vi "read_input_data.vi"(5 "Modulation info":T1={"Fs full"=0.0, "Fs high"=0.0, "Fs low"=0.0, "Read size"=5000, "FFT size low"=5000, "df low"=5000.0, "High carriers"=[], "Low carriers"=[], "Hi channels at low"=[7]} {"Hi channels at low" min=0 step=1; "Low carriers" format="%#_6p"; "High carriers" format="%#_6p"}, 7 "Config":T2={"IO params"={"Conversion"={"Rate"=4.0, "In channels"=2, "Out channels"=4}, "Carriers"={"Phase shift"=180.0, "Levels"=[[0.8, 0.8, 0.8], [0.03, 0.03, 0.03]], "Delay samples"=73.15}}, "High rate STFT"={"Win param"=101.5, "Window type"=61, "Win order"=2, "DFT size"=64, "Channels"=[7], "Oversample"=64}, "Low rate STFT"={"Win param"=120.0, "Window type"=61, "Win order"=8, "DFT size"=64, "Channels"=[7], "Oversample"=64}, "Filtering"={"Hum"={"Frequency"=0.0, "Tc"=0.0, "Limit"=101.5, "FFT filter"=FALSE, "Detrend mode"=enum."Robust linear", "Enable"=FALSE}, "Kalman"={"Process noise"=101.5, "Measure noise"=101.5, "Unlock m noise"=101.5, "Mode"=enum."FFT"}, "Distortion"={"LF cut"=101.5, "Tc"=3.0, "Limit"=101.5, "FFT filter"=FALSE, "Detrend mode"=enum."Robust linear", "Enable"=FALSE}, "Lowpass"={"Frequency"=0.0, "Order"=0, "Enable"=FALSE}, "Impulse"={"Win order"=102, "Locked limit"=101.5, "Locked count"=102, "Threshold Tc"=101.5, "Thresh sigmas"=101.5, "Thresh min"=101.5, "After"=0, "Detrend"=FALSE, "Enable"=FALSE}}} {"Filtering"."Impulse"."Thresh min" format="%#_3p"; "Filtering"."Impulse"."Threshold Tc" format="%#_3p"; "Filtering"."Impulse"."Locked limit" format="%#_3p"; "Filtering"."Impulse"."Thresh sigmas" format="%#_3p"; "Filtering"."Lowpass"."Frequency" format="%#_4p"; "Filtering"."Distortion"."Limit" format="%#_3p"; "Filtering"."Distortion"."LF cut" format="%#_3p"; "Filtering"."Kalman"."Unlock m noise" format="%#_3p"; "Filtering"."Kalman"."Measure noise" format="%#_3p"; "Filtering"."Kalman"."Process noise" format="%#_3p"; "Filtering"."Hum"."Limit" format="%#_3p"; "Filtering"."Hum"."Frequency" format="%#_4p"; "Low rate STFT"."Oversample" min=1 step=1; "Low rate STFT"."Channels" min=0 step=1; "Low rate STFT"."DFT size" min=1 step=1; "Low rate STFT"."Window type" items=["Rectangle"=0, "Hanning"=1, "Hamming"=2, "Blackman-Harris"=3, "Exact Blackman"=4, "Blackman"=5, "Flat Top"=6, "4 Term B-Harris "=7, "7 Term B-Harris"=8, "Low Sidelobe"=9, "Blackman Nuttall"=11, "Triangle"=30, "Bartlett-Hanning"=31, "Bohman"=32, "Parzen"=33, "Welch"=34, "Kaiser"=60, "Dolph-Chebyshev"=61, "Gaussian"=62]; "High rate STFT"."Oversample" min=1 step=1; "High rate STFT"."Channels" min=0 step=1; "High rate STFT"."DFT size" min=1 step=1; "High rate STFT"."Window type" items=["Rectangle"=0, "Hanning"=1, "Hamming"=2, "Blackman-Harris"=3, "Exact Blackman"=4, "Blackman"=5, "Flat Top"=6, "4 Term B-Harris "=7, "7 Term B-Harris"=8, "Low Sidelobe"=9, "Blackman Nuttall"=11, "Triangle"=30, "Bartlett-Hanning"=31, "Bohman"=32, "Parzen"=33, "Welch"=34, "Kaiser"=60, "Dolph-Chebyshev"=61, "Gaussian"=62]; "IO params"."Carriers"."Levels" min=0.0 step=0.1; "IO params"."Conversion"."Rate" format="%#_8g"}, 8 "error in":errorcluster, 9 "TCP channels":u32=3 min=1 max=12) -> (0 "error out":errorcluster, 1 "Data":i32[][](array[numeric]) format="%8x", 4 "TCP input":bool)   [LabVIEW 2014]
uses:
  ilemt_config.ctl
  IO_params.ctl
  stft_params.ctl
  <vilib>/Analysis/4window.llb/windowTd.ctl
  filter_params.ctl
  detrend_mode.ctl
  modulation_info.ctl
  ilemt_globals.vi
  <vilib>/Analysis/NI_AALPro.lvlib
panel:
  in  "Diff tag":u32 min=1 max=12
  in  "Same tag":u32 min=1 max=12
  out "Data size":i32[](array[numeric])
  out "length":i32
  in  "Timeouts":i32
  in  "Close count":i32
  out "error IO":errorcluster
  in  "TCP timeout ms":i32=5000
  # "Read the input data using TCP"
  # "Data read. Each row is data for one input channel.   Data is integer fraction of Bits/sample.  Eg. if bits/sample is 32, then data range is +/- 2^31, regardless of actual ADC resolution (in other words the data is low padded with zeros)."
  # "Number of channels to read"
  # "Did we read input from TCP?"
  # "Locals:"
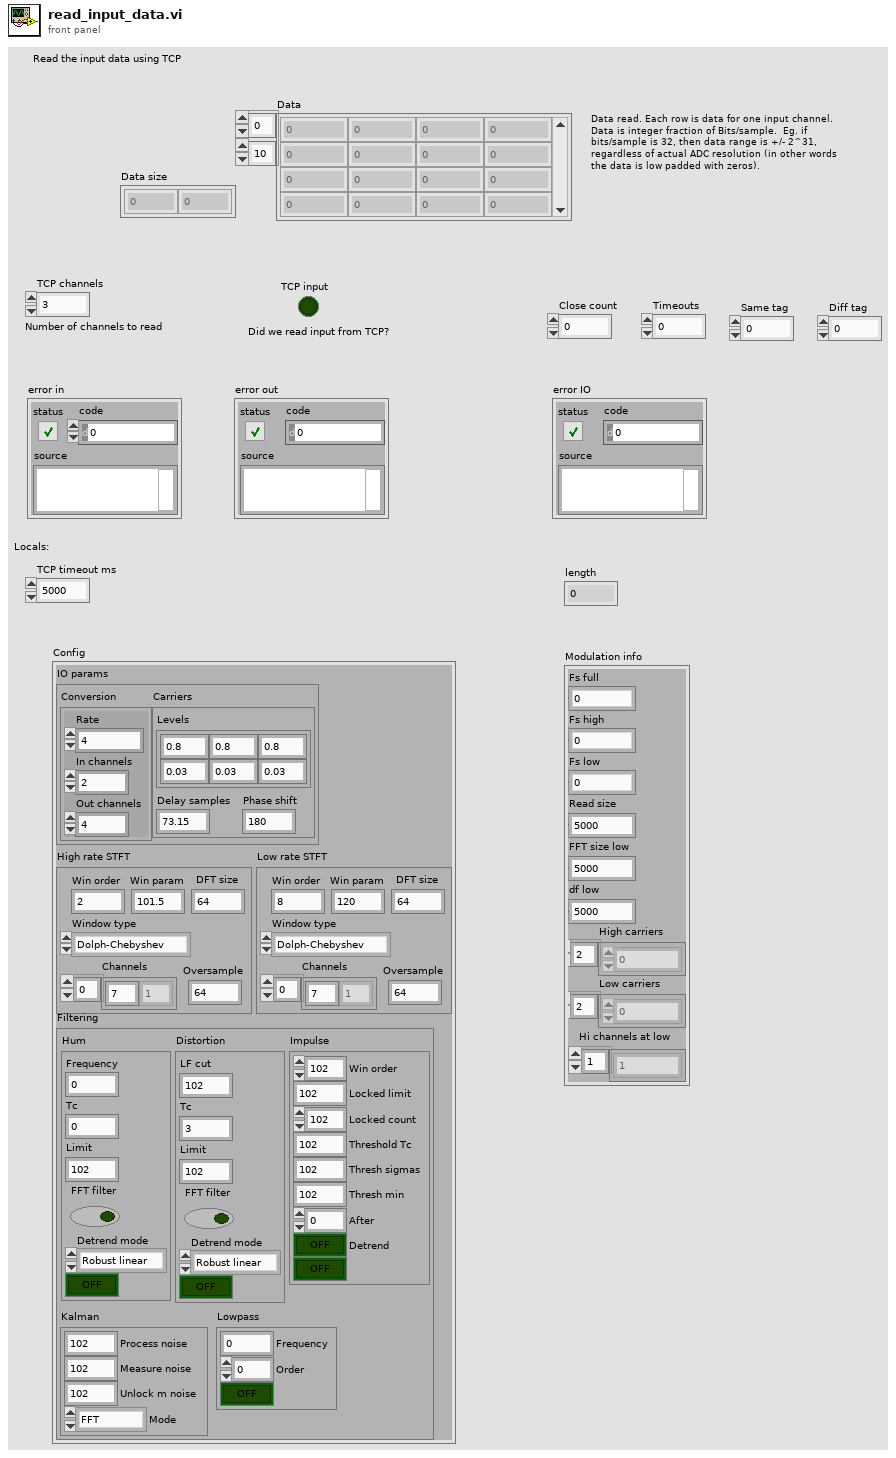
[diagram p1: front panel]
types:
  T1 = typedef "modulation_info.ctl" = cluster{"Fs full":dbl, "Fs high":dbl, "Fs low":dbl, "Read size":i32, "FFT size low":i32, "df low":dbl, "High carriers":dbl[], "Low carriers":dbl[], "Hi channels at low":i32[]}
  T2 = typedef "ilemt_config.ctl" = cluster{"IO params":T3, "High rate STFT":T4, "Low rate STFT":T4, "Filtering":T6}
  T3 = typedef "IO_params.ctl" = cluster{"Conversion":cluster{"Rate":dbl, "In channels":u32, "Out channels":u32}, "Carriers":cluster{"Phase shift":dbl, "Levels":dbl[][], "Delay samples":dbl}}
  T4 = typedef "stft_params.ctl" = cluster{"Win param":dbl, "Window type":T5, "Win order":i32, "DFT size":i32, "Channels":i32[], "Oversample":i32}
  T5 = typedef "NI_AALPro.lvlib/windowTd.ctl" = u32
  T6 = typedef "filter_params.ctl" = cluster{"Hum":cluster{"Frequency":dbl, "Tc":dbl, "Limit":dbl, "FFT filter":bool, "Detrend mode":T7, "Enable":bool}, "Kalman":cluster{"Process noise":dbl, "Measure noise":dbl, "Unlock m noise":dbl, "Mode":enum16{"FFT", "KF demod"}}, "Distortion":cluster{"LF cut":dbl, "Tc":dbl, "Limit":dbl, "FFT filter":bool, "Detrend mode":T7, "Enable":bool}, "Lowpass":cluster{"Frequency":dbl, "Order":i32, "Enable":bool}, "Impulse":cluster{"Win order":i32, "Locked limit":dbl, "Locked count":i32, "Threshold Tc":dbl, "Thresh sigmas":dbl, "Thresh min":dbl, "After":i32, "Detrend":bool, "Enable":bool}}
  T7 = typedef "detrend_mode.ctl" = enum16{"Zero mean", "Linear", "Robust linear"}
  T8 = enum16{"Standard", "Buffered", "CRLF", "Immediate"}
  T9 = enum16{"big-endian, network order", "native, host order", "little-endian"}
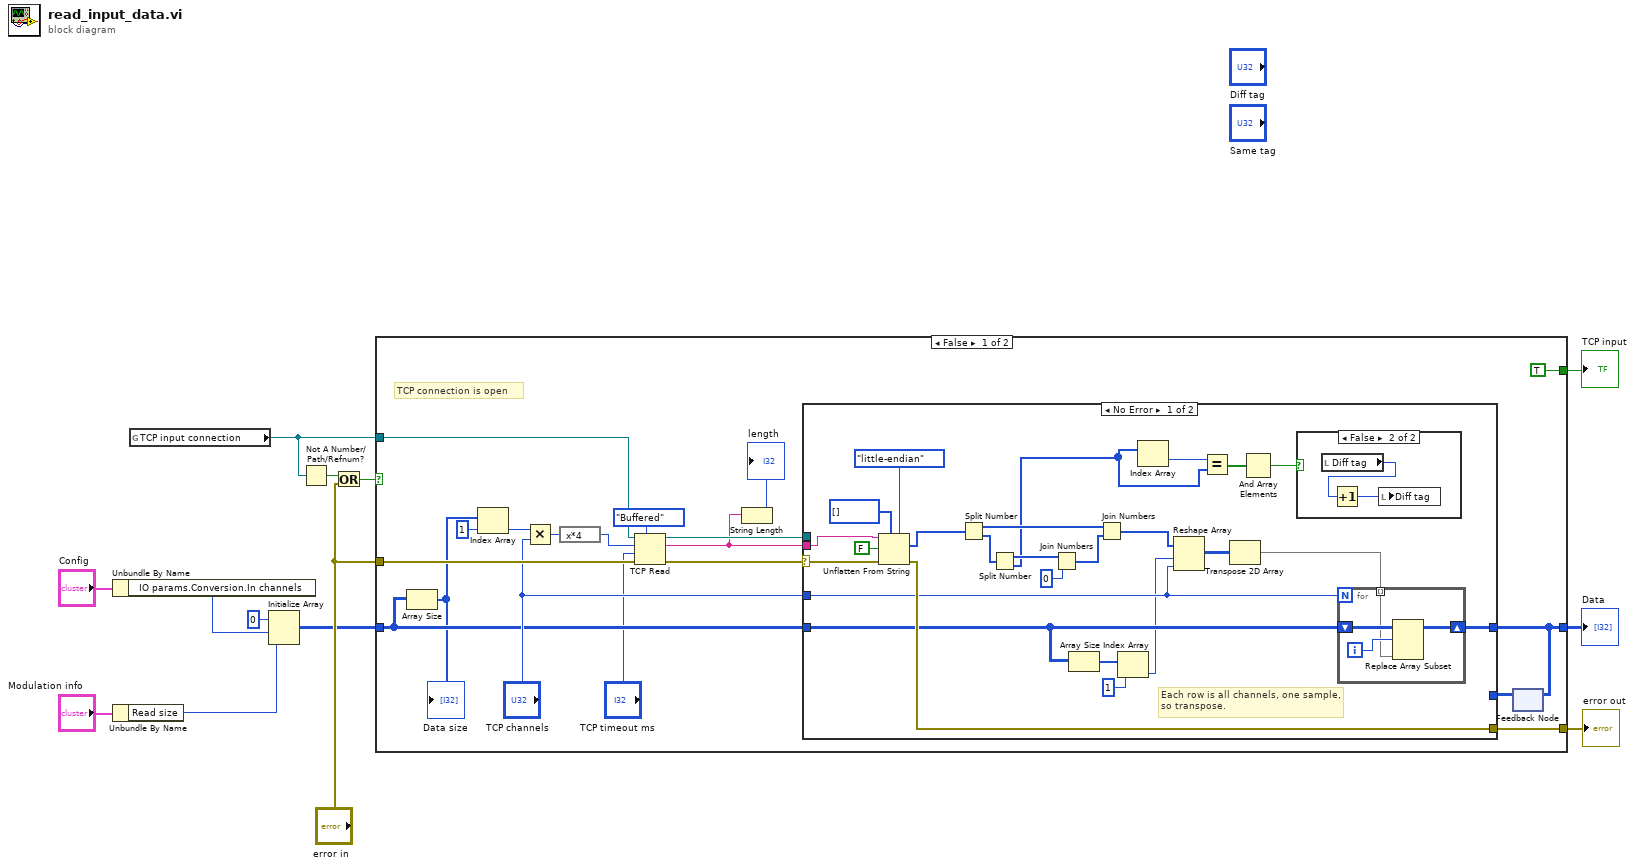
[diagram p0: block diagram]
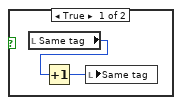
[diagram p2: hidden frame]
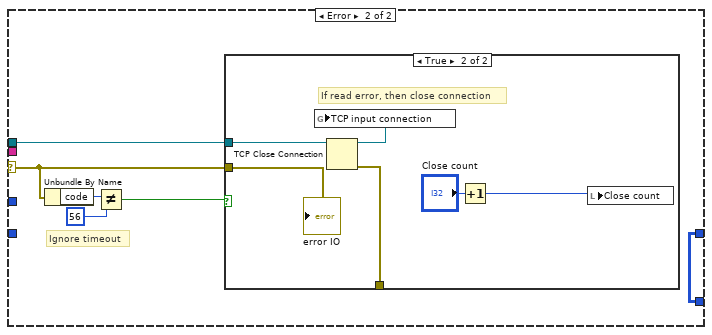
[diagram p3: hidden frame]
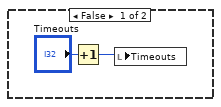
[diagram p4: hidden frame]
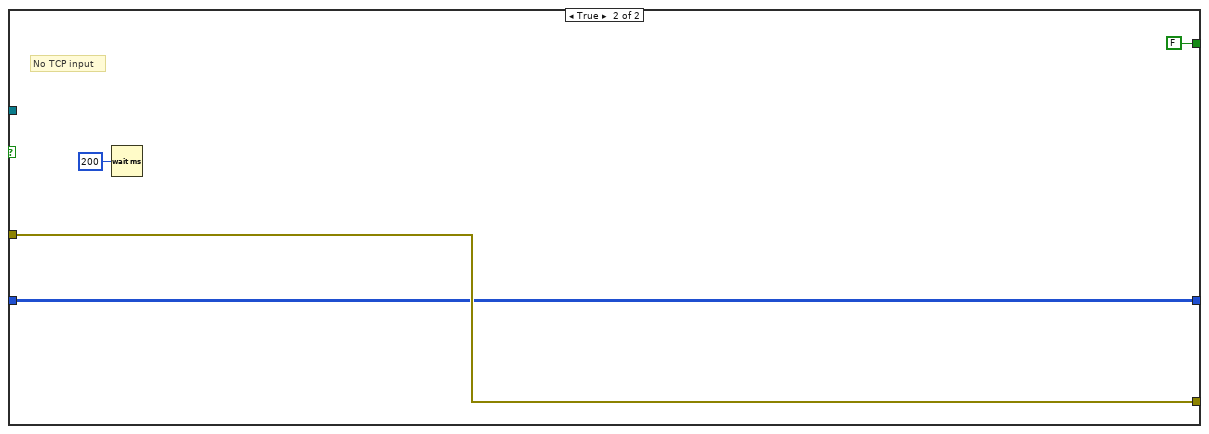
[diagram p5: hidden frame]
diagram:
  n1 = Unbundle By Name("Config") -> ("IO params.Conversion.In channels"=w2:u32)
  n2 = Unbundle By Name("Modulation info") -> ("Read size"=w1:i32)
  n3 = global read "ilemt_globals.vi" "TCP input connection"() -> (w11:refnum<k5>)
  n4 = Initialize Array(0 ("TCP channels"), w2, w1) -> (w4:i32[][])
  n5 = Not A Number/Path/Refnum?(number/path/refnum=w11) -> (NaN/Path/Refnum?=w8:bool)
  n6 = Or(x=w8, y="error in") -> (x .or. y?=w9:bool)
  n7 = case shown="False" w9 {
    tunnel: [w28 w83] -> w13
    tunnel: "error in" -> [w32 w83]
    tunnel: [w24 w82] -> w12
    tunnel: w4 -> [w22 w82]
    tunnel: w11 -> [w31 _]
    tunnel: [TRUE ("TCP input") FALSE ("TCP input")] -> w10
    frame False {
      # "TCP connection is open"
      n8 = Array Size(array=w22) -> (size(s)=w21:i32[])
      "Data size" <- w21
      n9 = Index Array(array=w21, index=1) -> (element=w19:i32)
      n10 = Multiply(x=w19, y="TCP channels") -> (x*y=w18:u32)
      n11 = expression code="x*4"(w18) -> (w17:u32)
      n12 = TCP Read(connection ID=w31, bytes to read=w17, error in (no error)=w32, 7:T8."Buffered" ("mode (standard)"), 9:"TCP timeout ms") -> (connection ID out=w26:refnum<k5>, data out=w15:string, error out=w27:errorcluster)
      n13 = String Length(string=w15) -> (length=→"length":i32)
      n14 = feedback #1() -> (w23:i32[][])  [unwired: 1 in]
      n15 = case shown="No Error" w27 {
        selector: w27 -> [w54 w70]
        tunnel: w22 -> [w50 _]
        tunnel: [w57 w66] -> w24
        tunnel: [w56 _] -> w28
        tunnel: w15 -> [w55 _]
        tunnel: w26 -> [_ w71]
        tunnel: "TCP channels" -> [w47 _]
        tunnel: w23 -> [_ w66]
        frame No Error {
          # "Each row is all channels, one sample,  so transpose."
          n16 = Unflatten From String(type=i32[] [] ("size(s)"), binary string=w55, data includes array or string size? (T)=FALSE, byte order (0:big-endian, network order)=T9."little-endian", error in (no error)=w54) -> (value=w33:i32[], error out=w56:errorcluster)  [unwired: 1 out]
          n17 = Split Number(x=w33) -> (hi(x)=w42:u16[], lo(x)=w43:u16[])
          n18 = Split Number(x=w43) -> (hi(x)=w40:u8[], lo(x)=w36:u8[])
          n19 = Join Numbers(hi=w40, lo=u8 0 ("index")) -> ((hi.lo)=w41:u16[])
          n20 = Array Size(array=w50) -> (size(s)=w49:i32[])
          n21 = Join Numbers(hi=w42, lo=w41) -> ((hi.lo)=w38:u32[])
          n22 = Index Array(array=w49, index=1) -> (element=w46:i32)
          n23 = Index Array(array=w36) -> (element=w37:u8)  [unwired: 1 in]
          n24 = Reshape Array(w38, w46, w47) -> (w45:u32[][])
          n25 = Equal?(x=w37, y=w36) -> (x = y?=w35:bool[])
          n26 = Transpose 2D Array(2D array=w45) -> (transposed array=w44:u32[][])
          n27 = And Array Elements(Boolean array=w35) -> (logical AND=w34:bool)
          n28 = case shown="False" w34 {
            frame True {
              n29 = local read "Same tag"() -> (w59:u32)
              n30 = Increment(x=w59) -> (x+1=w58:u32)
              n31 = local write "Same tag"(w58) -> ()
            }
            frame False {
              n32 = local read "Diff tag"() -> (w61:u32)
              n33 = Increment(x=w61) -> (x+1=w60:u32)
              n34 = local write "Diff tag"(w60) -> ()
            }
          }
          n35 = for {
            N: w47 -> [_]
            shift-right: [w64] -> w57
            shift-left: w50 -> [w65]
            tunnel: w44 -> [w62] mode=indexing
            i -> [w63]
            n36 = Replace Array Subset(array=w65, new element=w62, index (row)=w63) -> (w64:i32[][])  [unwired: 1 in]
          }
        }
        frame Error {
          # "Ignore timeout"
          n37 = Unbundle By Name(w70) -> ("code"=w69:i32)
          n38 = Not Equal?(x=w69, y=56) -> (x != y?=w67:bool)
          n39 = case shown="True" w67 {
            tunnel: w71 -> [_ w79]
            tunnel: [_ w77] -> _
            tunnel: w70 -> [_ w74]
            frame False {
              n40 = Increment(x="Timeouts") -> (x+1=w72:i32)
              n41 = local write "Timeouts"(w72) -> ()
            }
            frame True {
              # "If read error, then close connection"
              n42 = TCP Close Connection(connection ID=w79) -> (connection ID out=w78:refnum<k5>, error out=w77:errorcluster)  [unwired: 2 in]
              n43 = global write "ilemt_globals.vi" "TCP input connection"(w78) -> ()
              n44 = Increment(x="Close count") -> (x+1=w75:i32)
              n45 = local write "Close count"(w75) -> ()
              "error IO" <- w74
            }
          }
        }
      }
      n46 = feedback-in #1(w24) -> ()
    }
    frame True {
      # "No TCP input"
      n47 = Wait (ms)(milliseconds to wait=u32 200) -> ()  [unwired: 1 out]
    }
  }
  "Data" <- w12
  "error out" <- w13
  "TCP input" <- w10
